vi "Pulse Gen Control Panel (No Objects).vi"(8 "error in (no error)":errorcluster) -> (0 "error out":errorcluster)   [LabVIEW 2009]
uses:
  Global/GPIB Numbers.vi
  Pulse Generator.lvclass
panel:
  in  "Width/Duty\nUP/DOWN Ch2":bool
  in  "Width/Duty\nUP/DOWN Ch1":bool
  in  "Clear Error":bool
  out "Ready when \nblinking":bool
  in  "Copy actual to set":bool
  out "Pulse Mode":enum16{"Pulses", "Pattern"}(ring)
  out "Arming (Trigger) Source":T1(ring)
  in  "Populate fields with member data":bool
  out "Strobe Pattern":string
  in  "Strobe Pattern Set":string
  out "StrobeDataBuffer":digitalwaveform(graph)
  in  "Enable/disable":bool
  in  "Modes (changes immediately)":T2(radio)
  in  "BitPeriodSet":dbl[unit]
  out "BitPeriod":dbl[unit]
  out "Ch2Pattern":string
  in  "Ch2Pattern Set":string
  out "Ch1Pattern":string
  in  "Set Patterns":bool
  in  "Ch1Pattern Set":string
  in  "Ch2Duty (%) Set":dbl=10.0
  in  "Ch1Duty (%) Set":dbl=10.0
  in  "Ch1Delay Set":dbl[unit]
  in  "Ch2Delay Set":dbl[unit]
  in  "stop":bool
  out "Ch1DataBuffer":digitalwaveform(graph)
  out "Ch2DataBuffer":digitalwaveform(graph)
  in  "Ch2 Sync":bool
  in  "Ch1 Sync":bool
  in  "Ch2 Toggle":bool
  in  "Ch1 NOT Toggle":bool
  in  "Ch1 Toggle":bool
  in  "Ch2 NOT Toggle":bool
  in  "OverallPeriodSet":dbl[unit]
  in  "Ch2WidthSet":dbl[unit]=1e-09
  in  "Ch1WidthSet":dbl[unit]=1e-09
  in  "Ch2LowSet":dbl[unit]
  in  "Ch2HighSet":dbl[unit]
  in  "Ch1LowSet":dbl[unit]
  in  "Ch1HighSet":dbl[unit]
  in  "OverallFreqSet":dbl[unit]
  in  "Read to Control":bool
  in  "Set":bool
  out "Ch2Duty (%)":dbl
  out "Ch1Duty (%)":dbl
  out "Ch1Delay":dbl[unit]
  out "Ch2Delay":dbl[unit]
  out "Ch1Low":dbl[unit]
  out "Ch1High":dbl[unit]
  out "Ch2Width":dbl[unit]
  out "Ch1Width":dbl[unit]
  out "OverallPeriod":dbl[unit]
  out "Ch2Low":dbl[unit]
  out "Ch2High":dbl[unit]
  in  "Read":bool
  out "OverallFreq":dbl[unit]
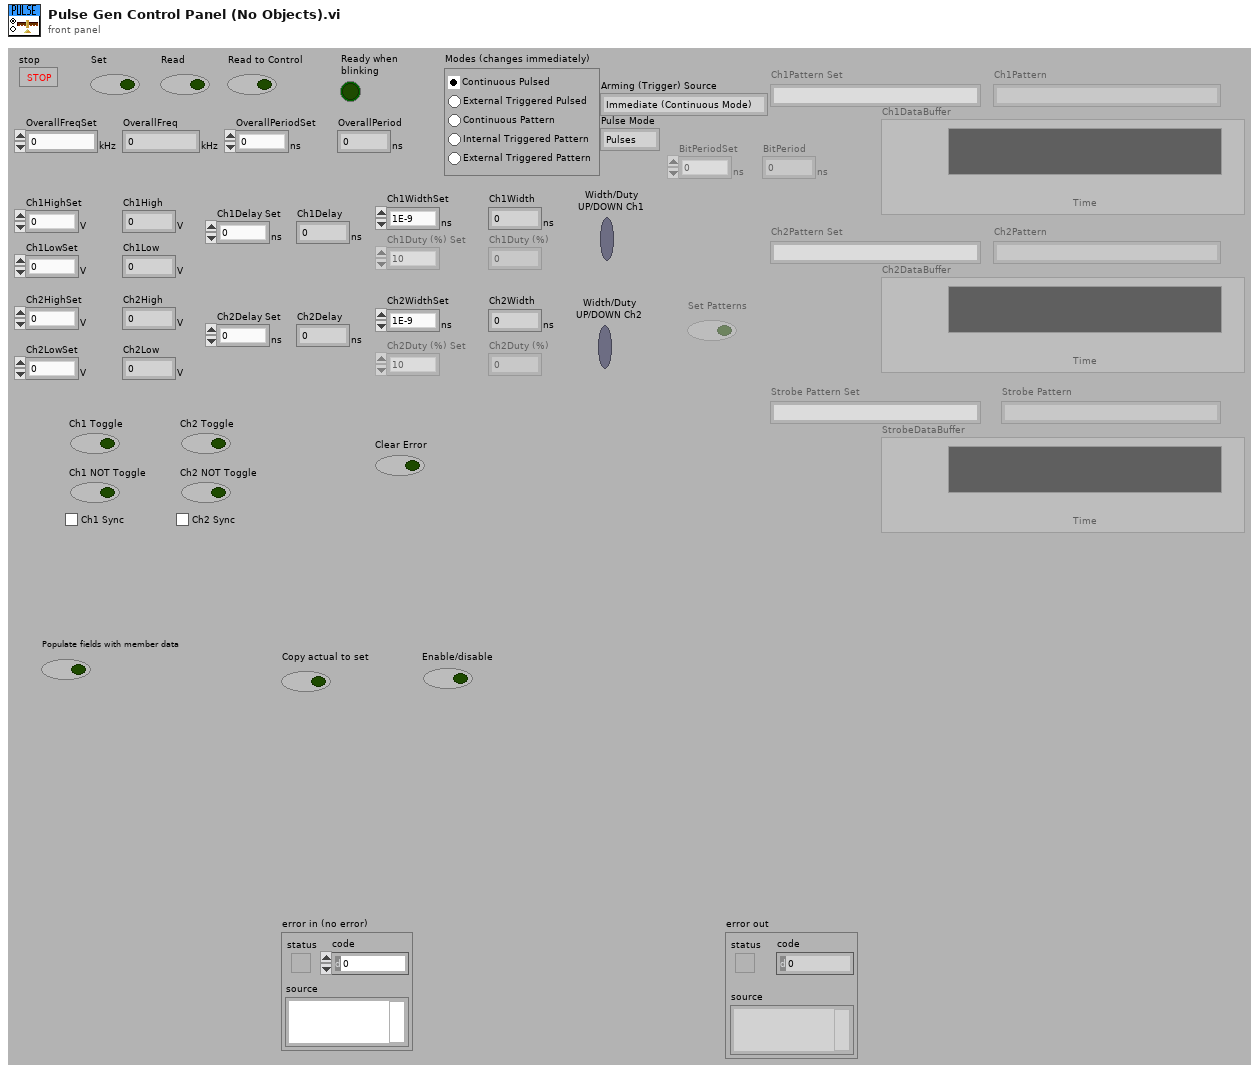
[diagram p1: front panel]
types:
  T1 = enum16{"Immediate (Continuous Mode)", "Internal PLL", "External", "Manual"}
  T2 = enum32{"Continuous Pulsed", "Continuous Pattern", "Internal Triggered Pattern", "External Triggered Pulsed", "External Triggered Pattern", "Other"}
  T3 = cluster{"Arming (Trigger) Source":u16, "Pulse Mode":u16, "Overall Period":dbl[unit], "Ch1Delay":dbl[unit], "Ch1Width":dbl[unit], "Ch2Delay":dbl[unit], "Ch2Width":dbl[unit], "Output Levels":cluster{"1 High":dbl[unit], "1 Low":dbl[unit], "2 High":dbl[unit], "2 Low":dbl[unit]}, "Outputs 1/!1/2/!2 ":bool[], "Bit Period":dbl[unit], "Ch1 Pattern":string, "Ch2 Pattern":string, "Strobe Pattern":string, "Ch1Width(true)":bool, "Ch2Width(true)":bool}
  T4 = typedef "GPIB Type Def.ctl" = cluster{"Name":string, "bus":dbl, "GPIB":dbl, "GPIB as string":string, "byte":i32, "VISA Resource Name":refnum<visa-resource-name>}
  T5 = enum16{"Internal Oscillator", "Internal PLL", "External Clock "}
  T6 = enum16{"Internal Oscillator", "Internal PLL", "Clock Input"}
  T7 = enum16{"Channel All ", "Channel 1", "Channel 2", "Channel 3", "Channels Combined"}
  T8 = cluster{"1 High":dbl[unit], "1 Low":dbl[unit], "2 High":dbl[unit], "2 Low":dbl[unit]}
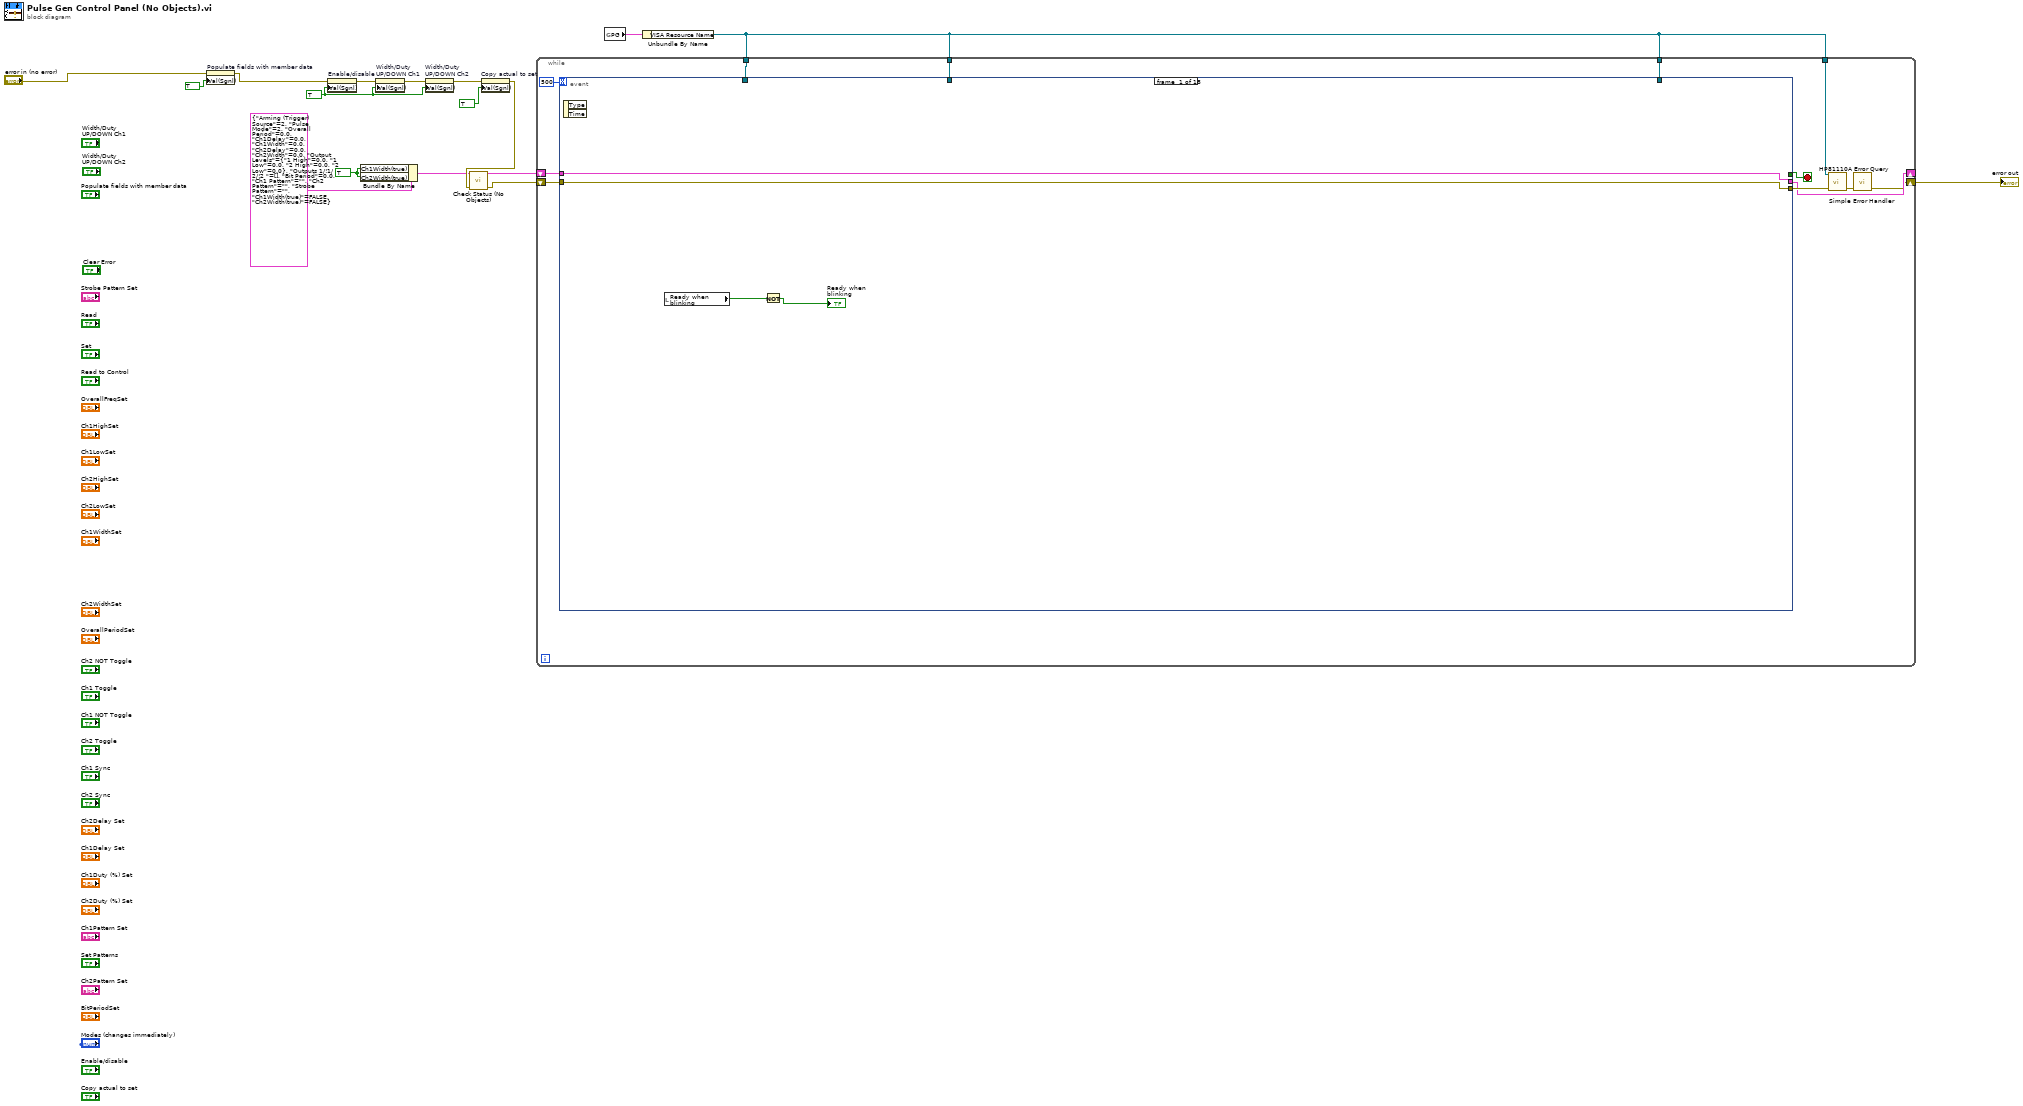
[diagram p0: block diagram]
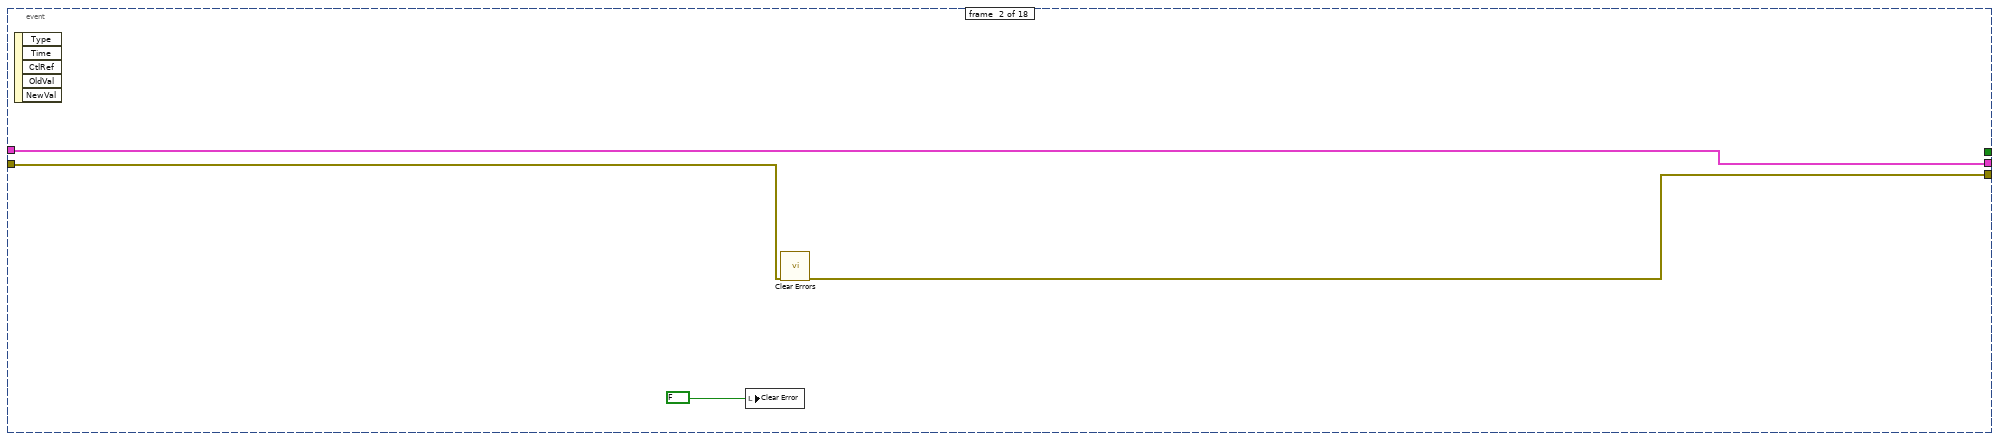
[diagram p2: hidden frame]
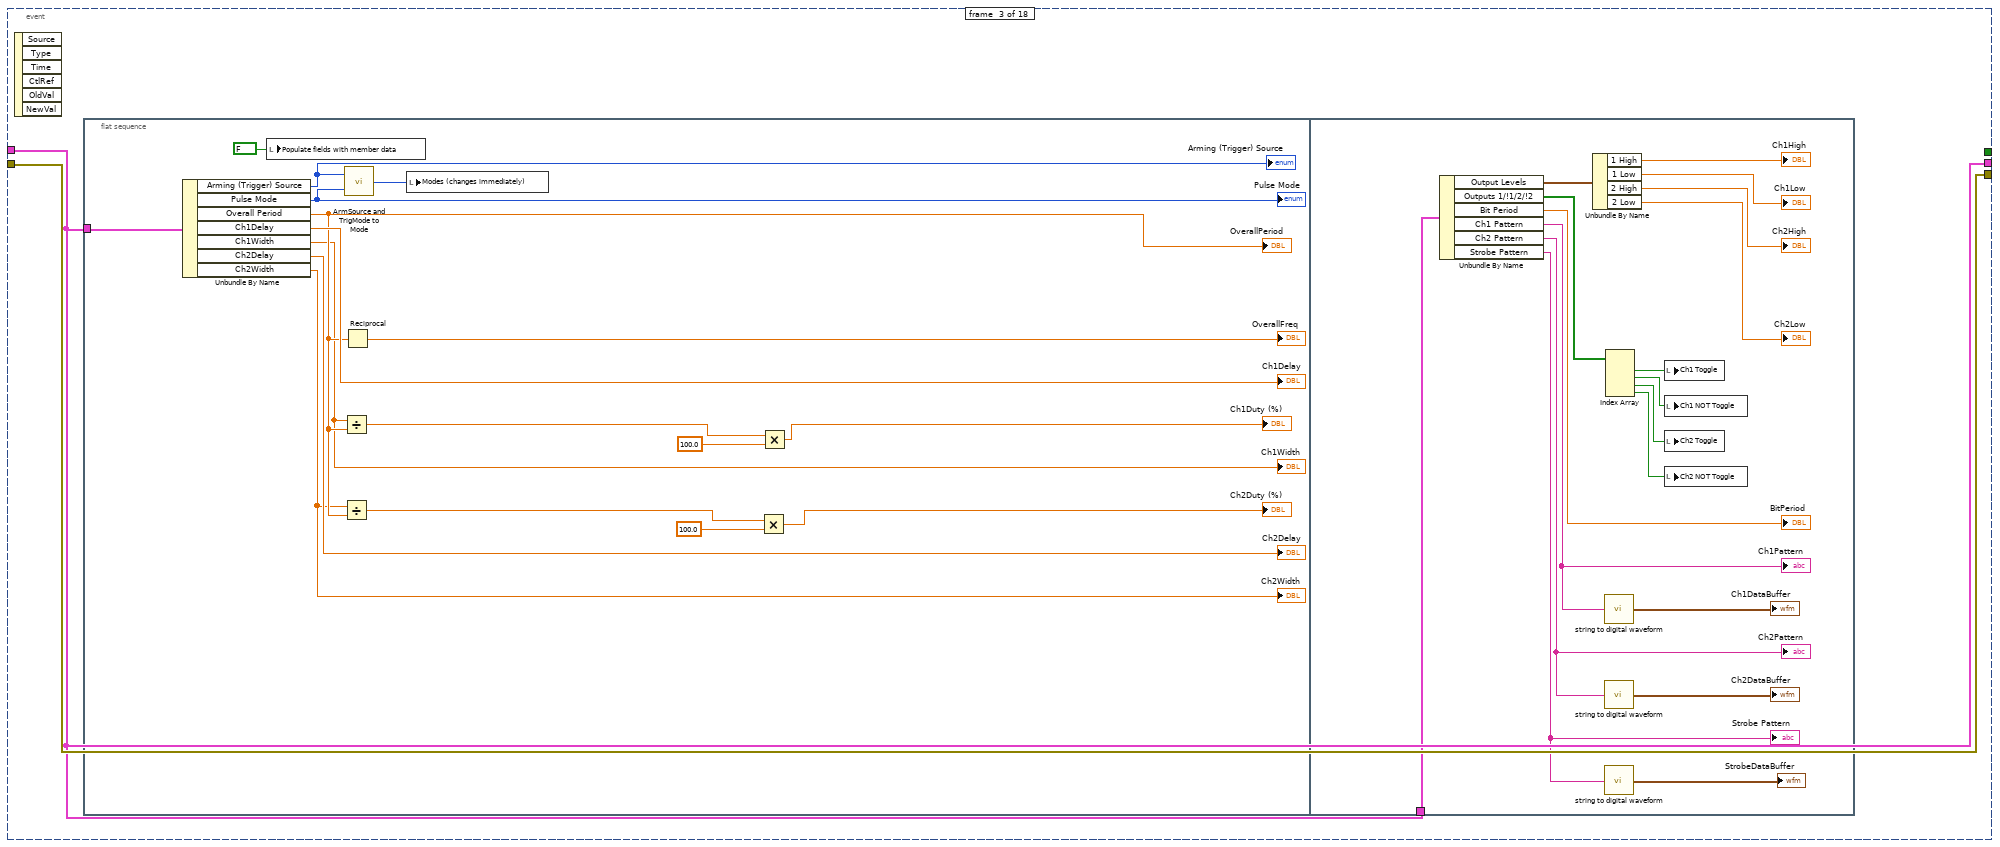
[diagram p3: hidden frame]
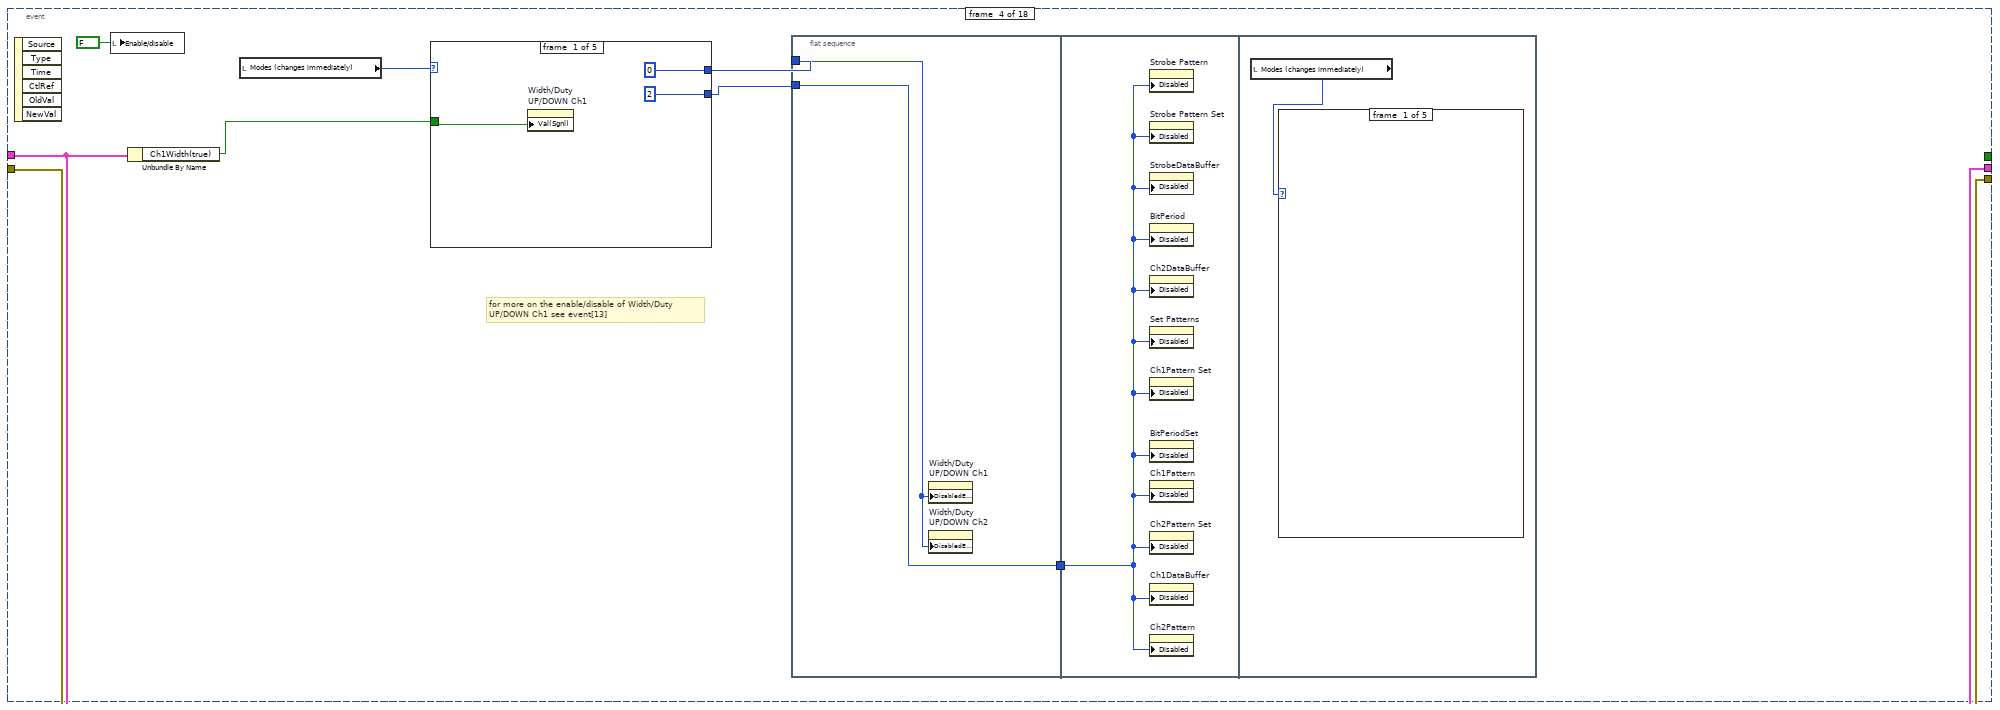
[diagram p4: hidden frame]
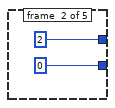
[diagram p5: hidden frame]
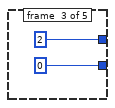
[diagram p6: hidden frame]
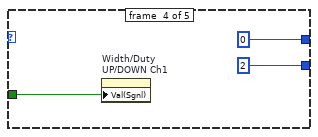
[diagram p7: hidden frame]
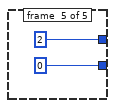
[diagram p8: hidden frame]
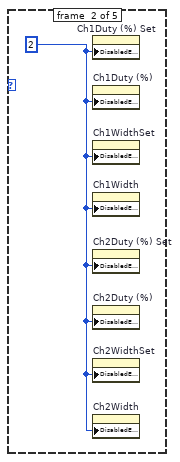
[diagram p9: hidden frame]
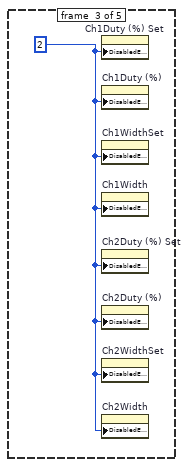
[diagram p10: hidden frame]
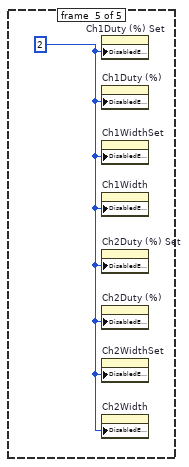
[diagram p12: hidden frame]
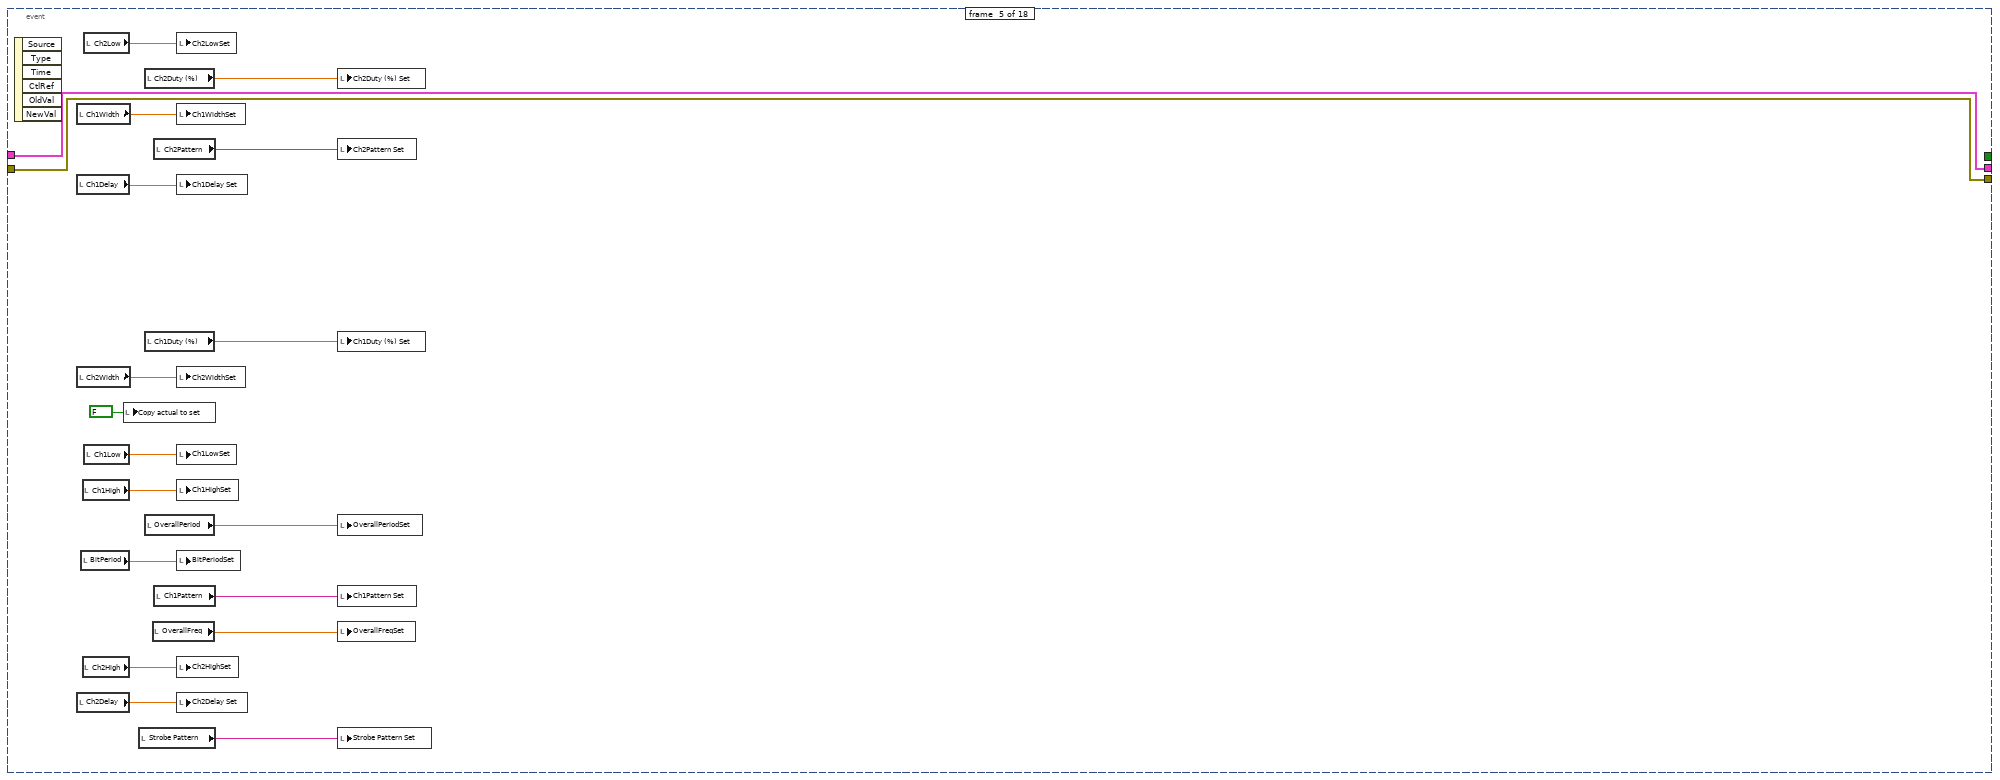
[diagram p13: hidden frame]
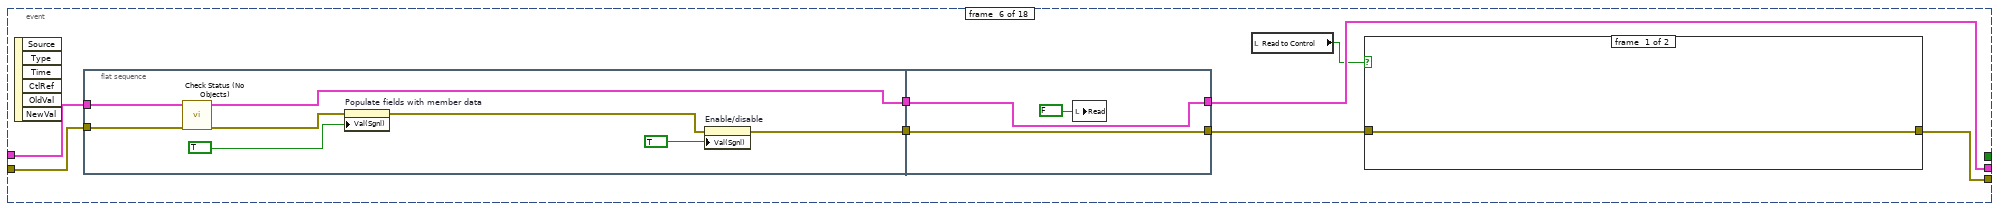
[diagram p14: hidden frame]
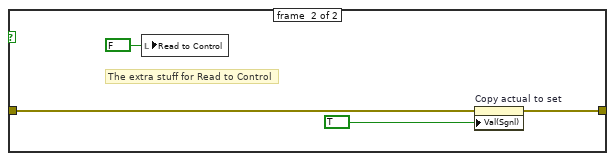
[diagram p15: hidden frame]
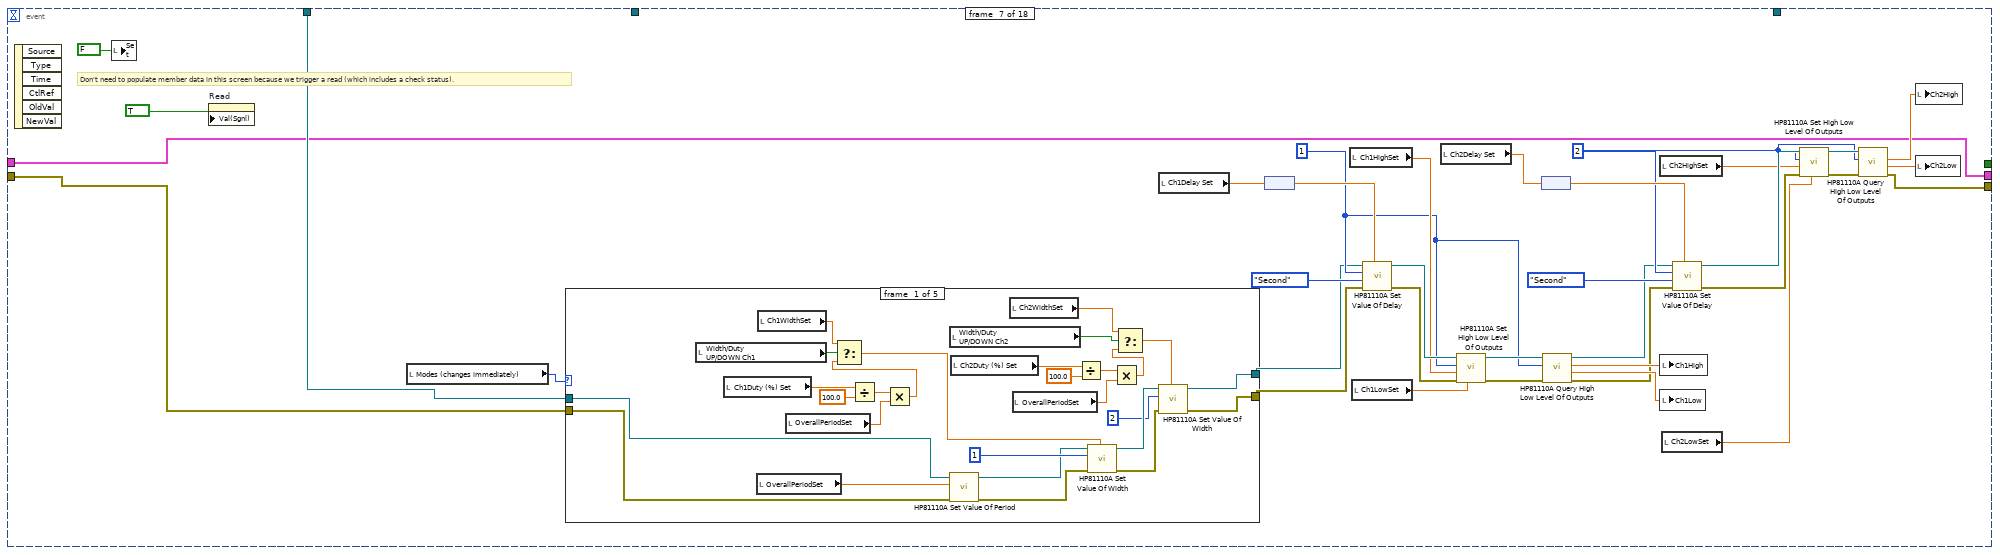
[diagram p16: hidden frame]
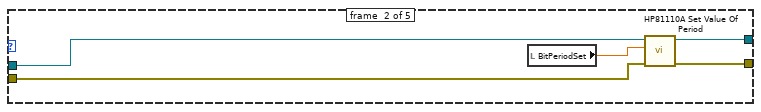
[diagram p17: hidden frame]
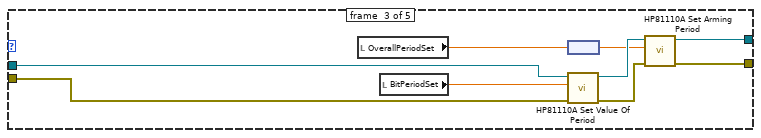
[diagram p18: hidden frame]
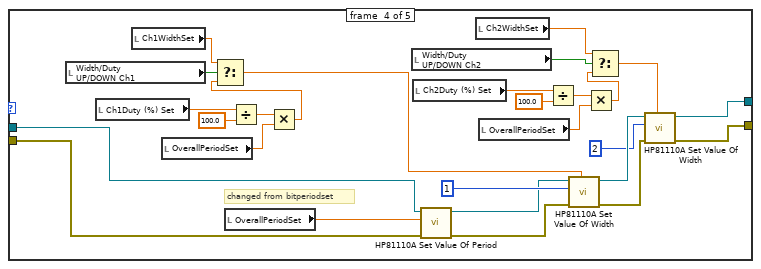
[diagram p19: hidden frame]
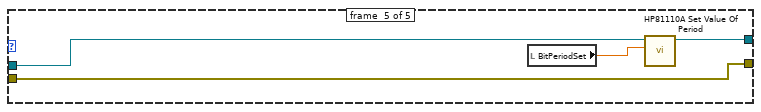
[diagram p20: hidden frame]
diagram:
  w10 = TRUE
  w11 = TRUE ("Value (Signaling)")
  n1 = property on="Populate fields with member data" class="Bool (strict)"(error in="error in (no error)", "Val(Sgnl)"=TRUE ("Value (Signaling)")) -> (error out=w15:errorcluster)  [unwired: 1 in, 1 out]
  n2 = property on="Enable/disable" class="Bool (strict)"(error in=w15, "Val(Sgnl)"=w11) -> (error out=w14:errorcluster)  [unwired: 1 in, 1 out]
  n3 = Bundle By Name(cluster=T3 {"Arming (Trigger) Source"=2, "Pulse Mode"=2, "Overall Period"=0.0, "Ch1Delay"=0.0, "Ch1Width"=0.0, "Ch2Delay"=0.0, "Ch2Width"=0.0, "Output Levels"={"1 High"=0.0, "1 Low"=0.0, "2 High"=0.0, "2 Low"=0.0}, "Outputs 1/!1/2/!2 "=[], "Bit Period"=0.0, "Ch1 Pattern"="", "Ch2 Pattern"="", "Strobe Pattern"="", "Ch1Width(true)"=FALSE, "Ch2Width(true)"=FALSE} ("Cluster of class private data"), "Ch1Width(true)"=w10, "Ch2Width(true)"=w10) -> (w1:T3)
  n4 = property on="Width/Duty\nUP/DOWN Ch1" class="Bool (strict)"(error in=w14, "Val(Sgnl)"=w11) -> (error out=w12:errorcluster)  [unwired: 1 in, 1 out]
  n5 = property on="Width/Duty\nUP/DOWN Ch2" class="Bool (strict)"(error in=w12, "Val(Sgnl)"=w11) -> (error out=w13:errorcluster)  [unwired: 1 in, 1 out]
  n6 = property on="Copy actual to set" class="Bool (strict)"(error in=w13, "Val(Sgnl)"=TRUE ("Value (Signaling)")) -> (error out=w4:errorcluster)  [unwired: 1 in, 1 out]
  n7 = call "Check Status (No Objects).vi"("error in (no error)"=w4, "Cluster In"=w1) -> ("error out"=w3:errorcluster, "Cluster Out"=w2:T3)  [unwired: 6 in, 2 out]
  n8 = global read "GPIB Numbers.vi" "PG"() -> (w7:T4)
  n9 = Unbundle By Name(w7) -> ("VISA Resource Name"=w5:refnum<visa-resource-name>)
  n10 = while {
    shift-right: [w22] -> _
    shift-left: w2 -> [w27]
    shift-right: [w18] -> w6
    shift-left: w3 -> [w26]
    tunnel: w5 -> [w24]
    tunnel: w5 -> [w21]
    tunnel: w5 -> [w20]
    tunnel: w5 -> [w19]
    stop <- w29 stop-if-true
    n11 = event shown="[5] \"Read\", \"Read to Control\": Value Change" {
      selector: _ -> [_ _ _ _ _ _ _ _ _ _ _ _ _ _ _ _ _ _]
      dyn-events: _ -> [_ _ _ _ _ _ _ _ _ _ _ _ _ _ _ _ _ _]
      timeout: 500 -> [_ _ _ _ _ _ _ _ _ _ _ _ _ _ _ _ _ _]
      tunnel: [_ _ _ _ _ _ _ _ _ _ _ _ "stop" _ _ _ _ _] -> w29
      tunnel: w26 -> [w32 w37 w39 w81 w103 w128 w147 w252 w280 w295 w314 w337 w350 w370 w372 w382 w392 w398]
      tunnel: [w32 w35 w39 w81 w103 w124 w146 w254 w282 w294 w314 w337 w350 w370 w372 w382 w392 w398] -> w23
      tunnel: w27 -> [w33 w36 w38 w76 w104 w127 w145 w253 w281 w293 w315 w338 w349 w357 w371 w381 w391 w399]
      tunnel: [w33 w36 w38 w76 w104 w126 w145 w253 w281 w302 w315 w338 w349 w356 w371 w381 w391 w399] -> w22
      tunnel: w21 -> [_ _ _ _ _ _ w148 _ _ _ _ _ _ _ _ _ _ _]
      tunnel: w20 -> [_ _ _ _ _ _ _ w255 w279 _ _ _ _ _ _ _ _ _]
      tunnel: w19 -> [_ _ _ _ _ _ _ _ _ w296 _ _ _ _ _ _ _ _]
      event #0 {
        n12 = event-data() -> ()  [unwired: 3 out]
        n13 = local read "Ready when \nblinking"() -> (w31:bool)
        n14 = Not(x=w31) -> (.not. x?=→"Ready when \nblinking":bool)
      }
      event #1 {
        n15 = event-data() -> ()  [unwired: 6 out]
        n16 = local write "Clear Error"(FALSE ("Clear Error")) -> ()
        n17 = call <vilib>:"Clear Errors.vi"("error in (no error)"=w37) -> ("error out"=w35:errorcluster)  [unwired: 6 in]
      }
      event #2 {
        n18 = event-data() -> ()  [unwired: 7 out]
        n19 = flat-sequence {
          tunnel: w38 -> [w46]
          tunnel: w38 -> [w57]
          frame #0 {
            n20 = Unbundle By Name(w46) -> ("Arming (Trigger) Source"=w49:u16, "Pulse Mode"=w48:u16, "Overall Period"=w52:dbl[unit], "Ch1Delay"=→"Ch1Delay":dbl[unit], "Ch1Width"=w51:dbl[unit], "Ch2Delay"=→"Ch2Delay":dbl[unit], "Ch2Width"=w50:dbl[unit])
            "OverallPeriod" <- w52
            "Ch1Width" <- w51
            "Ch2Width" <- w50
            "Arming (Trigger) Source" <- w49
            "Pulse Mode" <- w48
            n21 = local write "Populate fields with member data"(FALSE ("Populate fields with member data")) -> ()
            n22 = Divide(x=w51, y=w52) -> (x/y=w43:dbl)
            n23 = Divide(x=w50, y=w52) -> (x/y=w41:dbl)
            n24 = Reciprocal(x=w52) -> (1/x=→"OverallFreq":dbl[unit])
            n25 = call "ArmSource and TrigMode to Mode.vi"("Pulse Mode"=w48, "Arming (Trigger) Source (0:Internal PLL)"=w49) -> ("Modes (changes immediately)"=w47:T2)
            n26 = local write "Modes (changes immediately)"(w47) -> ()
            n27 = Multiply(x=w41, y=100.0) -> (x*y=→"Ch2Duty (%)":dbl)
            n28 = Multiply(x=w43, y=100.0) -> (x*y=→"Ch1Duty (%)":dbl)
          }
          frame #1 {
            n29 = Unbundle By Name(w57) -> ("Output Levels"=w69:T8, "Outputs 1/!1/2/!2"=w70:bool[], "Bit Period"=→"BitPeriod":dbl[unit], "Ch1 Pattern"=w72:string, "Ch2 Pattern"=w73:string, "Strobe Pattern"=w74:string)
            "Ch1Pattern" <- w72
            "Ch2Pattern" <- w73
            "Strobe Pattern" <- w74
            n30 = Unbundle By Name(w69) -> ("1 High"=→"Ch1High":dbl[unit], "1 Low"=→"Ch1Low":dbl[unit], "2 High"=→"Ch2High":dbl[unit], "2 Low"=→"Ch2Low":dbl[unit])
            n31 = call "string to digital waveform.vi"("String"=w72) -> ("digital waveform"=→"Ch1DataBuffer":digitalwaveform)
            n32 = call "string to digital waveform.vi"("String"=w73) -> ("digital waveform"=→"Ch2DataBuffer":digitalwaveform)
            n33 = call "string to digital waveform.vi"("String"=w74) -> ("digital waveform"=→"StrobeDataBuffer":digitalwaveform)
            n34 = Index Array(array=w70) -> (element #1=w65:bool, element #2=w66:bool, element #3=w67:bool, element #4=w68:bool)  [unwired: 4 in]
            n35 = local write "Ch1 Toggle"(w65) -> ()
            n36 = local write "Ch1 NOT Toggle"(w66) -> ()
            n37 = local write "Ch2 Toggle"(w67) -> ()
            n38 = local write "Ch2 NOT Toggle"(w68) -> ()
          }
        }
      }
      event #3 {
        # "for more on the enable/disable of Width/Duty\nUP/DOWN Ch1 see event[13]"
        n39 = event-data() -> ()  [unwired: 7 out]
        n40 = local write "Enable/disable"(FALSE ("Enable/disable")) -> ()
        n41 = Unbundle By Name(w76) -> ("Ch1Width(true)"=w75:bool)
        n42 = local read "Modes (changes immediately)"() -> (w79:T2)
        n43 = case shown="\"Internal Triggered Pattern\"" w79 {
          tunnel: [2 0 0 2 0] -> w77
          tunnel: [0 2 2 0 2] -> w78
          tunnel: w75 -> [w83 _ _ w90 _]
          frame #0 {
            n44 = property on="Width/Duty\nUP/DOWN Ch1" class="Bool (strict)"("Val(Sgnl)"=w83) -> ()  [unwired: 2 in, 2 out]
          }
          frame #1 {
          }
          frame #2 {
          }
          frame #3 {
            n45 = property on="Width/Duty\nUP/DOWN Ch1" class="Bool (strict)"("Val(Sgnl)"=w90) -> ()  [unwired: 2 in, 2 out]
          }
          frame #4 {
          }
        }
        n46 = flat-sequence {
          tunnel: [w96] -> w80
          tunnel: w78 -> [w95]
          tunnel: w77 -> [w96]
          tunnel: w80 -> [w97]
          frame #0 {
            n47 = property on="Width/Duty\nUP/DOWN Ch1" class="Bool (strict)"("DisabledEnum"=w95) -> ()  [unwired: 2 in, 2 out]
            n48 = property on="Width/Duty\nUP/DOWN Ch2" class="Bool (strict)"("DisabledEnum"=w95) -> ()  [unwired: 2 in, 2 out]
          }
          frame #1 {
            n49 = property on="Strobe Pattern" class="Str"("Disabled"=w97) -> ()  [unwired: 2 in, 2 out]
            n50 = property on="Strobe Pattern Set" class="Str"("Disabled"=w97) -> ()  [unwired: 2 in, 2 out]
            n51 = property on="StrobeDataBuffer" class="DigitalGraph (strict)"("Disabled"=w97) -> ()  [unwired: 2 in, 2 out]
            n52 = property on="BitPeriod" class="DigNum (strict)"("Disabled"=w97) -> ()  [unwired: 2 in, 2 out]
            n53 = property on="Ch2DataBuffer" class="DigitalGraph (strict)"("Disabled"=w97) -> ()  [unwired: 2 in, 2 out]
            n54 = property on="Set Patterns" class="Bool (strict)"("Disabled"=w97) -> ()  [unwired: 2 in, 2 out]
            n55 = property on="Ch1Pattern Set" class="Str"("Disabled"=w97) -> ()  [unwired: 2 in, 2 out]
            n56 = property on="BitPeriodSet" class="DigNum (strict)"("Disabled"=w97) -> ()  [unwired: 2 in, 2 out]
            n57 = property on="Ch1Pattern" class="Str"("Disabled"=w97) -> ()  [unwired: 2 in, 2 out]
            n58 = property on="Ch2Pattern Set" class="Str"("Disabled"=w97) -> ()  [unwired: 2 in, 2 out]
            n59 = property on="Ch1DataBuffer" class="DigitalGraph (strict)"("Disabled"=w97) -> ()  [unwired: 2 in, 2 out]
            n60 = property on="Ch2Pattern" class="Str"("Disabled"=w97) -> ()  [unwired: 2 in, 2 out]
          }
          frame #2 {
            n61 = local read "Modes (changes immediately)"() -> (w98:T2)
            n62 = case shown="\"External Triggered Pattern\"" w98 {
              frame #0 {
              }
              frame #1 {
                w99 = 2
                n63 = property on="Ch1Duty (%) Set" class="DigNum (strict)"("DisabledEnum"=w99) -> ()  [unwired: 2 in, 2 out]
                n64 = property on="Ch1Duty (%)" class="DigNum (strict)"("DisabledEnum"=w99) -> ()  [unwired: 2 in, 2 out]
                n65 = property on="Ch1WidthSet" class="DigNum (strict)"("DisabledEnum"=w99) -> ()  [unwired: 2 in, 2 out]
                n66 = property on="Ch1Width" class="DigNum (strict)"("DisabledEnum"=w99) -> ()  [unwired: 2 in, 2 out]
                n67 = property on="Ch2Duty (%) Set" class="DigNum (strict)"("DisabledEnum"=w99) -> ()  [unwired: 2 in, 2 out]
                n68 = property on="Ch2Duty (%)" class="DigNum (strict)"("DisabledEnum"=w99) -> ()  [unwired: 2 in, 2 out]
                n69 = property on="Ch2WidthSet" class="DigNum (strict)"("DisabledEnum"=w99) -> ()  [unwired: 2 in, 2 out]
                n70 = property on="Ch2Width" class="DigNum (strict)"("DisabledEnum"=w99) -> ()  [unwired: 2 in, 2 out]
              }
              frame #2 {
                w100 = 2
                n71 = property on="Ch1Duty (%) Set" class="DigNum (strict)"("DisabledEnum"=w100) -> ()  [unwired: 2 in, 2 out]
                n72 = property on="Ch1Duty (%)" class="DigNum (strict)"("DisabledEnum"=w100) -> ()  [unwired: 2 in, 2 out]
                n73 = property on="Ch1WidthSet" class="DigNum (strict)"("DisabledEnum"=w100) -> ()  [unwired: 2 in, 2 out]
                n74 = property on="Ch1Width" class="DigNum (strict)"("DisabledEnum"=w100) -> ()  [unwired: 2 in, 2 out]
                n75 = property on="Ch2Duty (%) Set" class="DigNum (strict)"("DisabledEnum"=w100) -> ()  [unwired: 2 in, 2 out]
                n76 = property on="Ch2Duty (%)" class="DigNum (strict)"("DisabledEnum"=w100) -> ()  [unwired: 2 in, 2 out]
                n77 = property on="Ch2WidthSet" class="DigNum (strict)"("DisabledEnum"=w100) -> ()  [unwired: 2 in, 2 out]
                n78 = property on="Ch2Width" class="DigNum (strict)"("DisabledEnum"=w100) -> ()  [unwired: 2 in, 2 out]
              }
              frame #3 {
              }
              frame #4 {
                w101 = 2
                n79 = property on="Ch1Duty (%) Set" class="DigNum (strict)"("DisabledEnum"=w101) -> ()  [unwired: 2 in, 2 out]
                n80 = property on="Ch1Duty (%)" class="DigNum (strict)"("DisabledEnum"=w101) -> ()  [unwired: 2 in, 2 out]
                n81 = property on="Ch1WidthSet" class="DigNum (strict)"("DisabledEnum"=w101) -> ()  [unwired: 2 in, 2 out]
                n82 = property on="Ch1Width" class="DigNum (strict)"("DisabledEnum"=w101) -> ()  [unwired: 2 in, 2 out]
                n83 = property on="Ch2Duty (%) Set" class="DigNum (strict)"("DisabledEnum"=w101) -> ()  [unwired: 2 in, 2 out]
                n84 = property on="Ch2Duty (%)" class="DigNum (strict)"("DisabledEnum"=w101) -> ()  [unwired: 2 in, 2 out]
                n85 = property on="Ch2WidthSet" class="DigNum (strict)"("DisabledEnum"=w101) -> ()  [unwired: 2 in, 2 out]
                n86 = property on="Ch2Width" class="DigNum (strict)"("DisabledEnum"=w101) -> ()  [unwired: 2 in, 2 out]
              }
            }
          }
        }
      }
      event #4 {
        n87 = event-data() -> ()  [unwired: 7 out]
        n88 = local read "Ch1Width"() -> (w116:dbl[unit])
        n89 = local read "Ch1Delay"() -> (w114:dbl[unit])
        n90 = local read "Ch2Width"() -> (w112:dbl[unit])
        n91 = local read "Ch2Delay"() -> (w110:dbl[unit])
        n92 = local read "BitPeriod"() -> (w106:dbl[unit])
        n93 = local read "Ch1High"() -> (w118:dbl[unit])
        n94 = local read "Ch2High"() -> (w109:dbl[unit])
        n95 = local read "Ch2Low"() -> (w113:dbl[unit])
        n96 = local read "Ch1Low"() -> (w117:dbl[unit])
        n97 = local write "Copy actual to set"(FALSE ("Copy actual to set")) -> ()
        n98 = local read "Strobe Pattern"() -> (w102:string)
        n99 = local read "Ch2Duty (%)"() -> (w111:dbl)
        n100 = local read "Ch1Duty (%)"() -> (w115:dbl)
        n101 = local read "OverallPeriod"() -> (w119:dbl[unit])
        n102 = local read "OverallFreq"() -> (w120:dbl[unit])
        n103 = local read "Ch2Pattern"() -> (w107:string)
        n104 = local read "Ch1Pattern"() -> (w108:string)
        n105 = local write "Ch2LowSet"(w113) -> ()
        n106 = local write "Ch1WidthSet"(w116) -> ()
        n107 = local write "Ch1Delay Set"(w114) -> ()
        n108 = local write "Ch2WidthSet"(w112) -> ()
        n109 = local write "Ch1LowSet"(w117) -> ()
        n110 = local write "Ch1HighSet"(w118) -> ()
        n111 = local write "BitPeriodSet"(w106) -> ()
        n112 = local write "Ch2HighSet"(w109) -> ()
        n113 = local write "Ch2Delay Set"(w110) -> ()
        n114 = local write "Ch2Duty (%) Set"(w111) -> ()
        n115 = local write "Ch2Pattern Set"(w107) -> ()
        n116 = local write "Ch1Duty (%) Set"(w115) -> ()
        n117 = local write "OverallPeriodSet"(w119) -> ()
        n118 = local write "Ch1Pattern Set"(w108) -> ()
        n119 = local write "OverallFreqSet"(w120) -> ()
        n120 = local write "Strobe Pattern Set"(w102) -> ()
      }
      event #5 {
        n121 = event-data() -> ()  [unwired: 7 out]
        n122 = flat-sequence {
          tunnel: w128 -> [w136]
          tunnel: w127 -> [w129]
          tunnel: [w135] -> w122
          tunnel: [w134] -> w121
          tunnel: [w138] -> w125
          tunnel: [w139] -> w126
          tunnel: w122 -> [w139]
          tunnel: w121 -> [w138]
          frame #0 {
            n123 = call "Check Status (No Objects).vi"("error in (no error)"=w136, "Cluster In"=w129) -> ("error out"=w131:errorcluster, "Cluster Out"=w135:T3)  [unwired: 6 in, 2 out]
            n124 = property on="Populate fields with member data" class="Bool (strict)"(error in=w131, "Val(Sgnl)"=TRUE ("Value (Signaling)")) -> (error out=w130:errorcluster)  [unwired: 1 in, 1 out]
            n125 = property on="Enable/disable" class="Bool (strict)"(error in=w130, "Val(Sgnl)"=TRUE ("Value (Signaling)")) -> (error out=w134:errorcluster)  [unwired: 1 in, 1 out]
          }
          frame #1 {
            n126 = local write "Read"(FALSE) -> ()
          }
        }
        n127 = local read "Read to Control"() -> (w123:bool)
        n128 = case shown="False" w123 {
          tunnel: w125 -> [w140 w142]
          tunnel: [w140 w141] -> w124
          frame #0 {
          }
          frame #1 {
            # "The extra stuff for Read to Control"
            n129 = local write "Read to Control"(FALSE) -> ()
            n130 = property on="Copy actual to set" class="Bool (strict)"(error in=w142, "Val(Sgnl)"=TRUE ("Value (Signaling)")) -> (error out=w141:errorcluster)  [unwired: 1 in, 1 out]
          }
        }
      }
      event #6 {
        w154 = 1
        w159 = 2
        # "Don't need to populate member data in this screen because we trigger a read (which includes a check status)."
        n131 = event-data() -> ()  [unwired: 7 out]
        n132 = local write "Set"(FALSE) -> ()
        n133 = property on="Read" class="Bool (strict)"("Val(Sgnl)"=TRUE ("Value (Signaling)")) -> ()  [unwired: 2 in, 2 out]
        n134 = local read "Modes (changes immediately)"() -> (w151:T2)
        n135 = case shown="\"External Triggered Pulsed\"" w151 {
          tunnel: w148 -> [w201 w210 w215 w221 w250]
          tunnel: w147 -> [w200 w208 w213 w240 w248]
          tunnel: [w197 w209 w214 w241 w249] -> w150
          tunnel: [w196 w207 w212 w238 w248] -> w149
          frame #0 {
            n136 = local read "Width/Duty\nUP/DOWN Ch1"() -> (w195:bool)
            n137 = local read "Ch1Duty (%) Set"() -> (w192:dbl)
            n138 = local read "OverallPeriodSet"() -> (w206:dbl[unit])
            n139 = local read "Ch1WidthSet"() -> (w194:dbl[unit])
            n140 = local read "OverallPeriodSet"() -> (w190:dbl[unit])
            n141 = Divide(x=w192, y=100.0) -> (x/y=w191:dbl)
            n142 = Multiply(x=w191, y=w190) -> (x*y=w189:dbl[unit])
            n143 = Select(t=w194, s=w195, f=w189) -> (s? t:f=w180:dbl[unit])
            n144 = local read "Width/Duty\nUP/DOWN Ch2"() -> (w183:bool)
            n145 = call "HP81110A Set Value Of Period.vi"("error in (no error)"=w200, "Period Value"=w206, "VISA session"=w201) -> ("error out"=w198:errorcluster, "dup VISA session"=w199:refnum<visa-resource-name>)  [unwired: 7 out]
            n146 = local read "Ch2Duty (%) Set"() -> (w186:dbl)
            n147 = local read "Ch2WidthSet"() -> (w182:dbl[unit])
            n148 = local read "OverallPeriodSet"() -> (w188:dbl[unit])
            n149 = Divide(x=w186, y=100.0) -> (x/y=w187:dbl)
            n150 = call "HP81110A Set Value Of Width.vi"("Width Value (100.0E-9)"=w180, "error in (no error)"=w198, "Channel (1:Channel 1)"=1, "VISA session"=w199) -> ("error out"=w205:errorcluster, "dup VISA session"=w204:refnum<visa-resource-name>)  [unwired: 1 in, 5 out]
            n151 = Multiply(x=w187, y=w188) -> (x*y=w184:dbl[unit])
            n152 = Select(t=w182, s=w183, f=w184) -> (s? t:f=w181:dbl[unit])
            n153 = call "HP81110A Set Value Of Width.vi"("Width Value (100.0E-9)"=w181, "error in (no error)"=w205, "Channel (1:Channel 1)"=2, "VISA session"=w204) -> ("error out"=w196:errorcluster, "dup VISA session"=w197:refnum<visa-resource-name>)  [unwired: 1 in, 5 out]
          }
          frame #1 {
            n154 = local read "BitPeriodSet"() -> (w211:dbl[unit])
            n155 = call "HP81110A Set Value Of Period.vi"("error in (no error)"=w208, "Period Value"=w211, "VISA session"=w210) -> ("error out"=w207:errorcluster, "dup VISA session"=w209:refnum<visa-resource-name>)  [unwired: 7 out]
          }
          frame #2 {
            n156 = local read "OverallPeriodSet"() -> (w217:dbl[unit])
            n157 = local read "BitPeriodSet"() -> (w216:dbl[unit])
            n158 = node(w217) -> (w218:dbl)
            n159 = call "HP81110A Set Value Of Period.vi"("error in (no error)"=w213, "Period Value"=w216, "VISA session"=w215) -> ("error out"=w220:errorcluster, "dup VISA session"=w219:refnum<visa-resource-name>)  [unwired: 7 out]
            n160 = call "HP81110A Set Arming Period.vi"("error in (no error)"=w220, "Period Value (10.0E-6 Sec)"=w218, "VISA session"=w219) -> ("error out"=w212:errorcluster, "dup VISA session"=w214:refnum<visa-resource-name>)  [unwired: 7 out]
          }
          frame #3 {
            # "changed from bitperiodset"
            n161 = local read "Width/Duty\nUP/DOWN Ch1"() -> (w237:bool)
            n162 = local read "Ch1Duty (%) Set"() -> (w234:dbl)
            n163 = local read "Ch1WidthSet"() -> (w236:dbl[unit])
            n164 = local read "OverallPeriodSet"() -> (w232:dbl[unit])
            n165 = local read "OverallPeriodSet"() -> (w243:dbl[unit])
            n166 = Divide(x=w234, y=100.0) -> (x/y=w233:dbl)
            n167 = Multiply(x=w233, y=w232) -> (x*y=w231:dbl[unit])
            n168 = Select(t=w236, s=w237, f=w231) -> (s? t:f=w224:dbl[unit])
            n169 = local read "Width/Duty\nUP/DOWN Ch2"() -> (w226:bool)
            n170 = local read "Ch2Duty (%) Set"() -> (w228:dbl)
            n171 = call "HP81110A Set Value Of Period.vi"("error in (no error)"=w240, "Period Value"=w243, "VISA session"=w221) -> ("error out"=w239:errorcluster, "dup VISA session"=w242:refnum<visa-resource-name>)  [unwired: 7 out]
            n172 = local read "Ch2WidthSet"() -> (w225:dbl[unit])
            n173 = local read "OverallPeriodSet"() -> (w230:dbl[unit])
            n174 = Divide(x=w228, y=100.0) -> (x/y=w229:dbl)
            n175 = call "HP81110A Set Value Of Width.vi"("Width Value (100.0E-9)"=w224, "error in (no error)"=w239, "Channel (1:Channel 1)"=1, "VISA session"=w242) -> ("error out"=w247:errorcluster, "dup VISA session"=w246:refnum<visa-resource-name>)  [unwired: 1 in, 5 out]
            n176 = Multiply(x=w229, y=w230) -> (x*y=w222:dbl[unit])
            n177 = Select(t=w225, s=w226, f=w222) -> (s? t:f=w223:dbl[unit])
            n178 = call "HP81110A Set Value Of Width.vi"("Width Value (100.0E-9)"=w223, "error in (no error)"=w247, "Channel (1:Channel 1)"=2, "VISA session"=w246) -> ("error out"=w238:errorcluster, "dup VISA session"=w241:refnum<visa-resource-name>)  [unwired: 1 in, 5 out]
          }
          frame #4 {
            n179 = local read "BitPeriodSet"() -> (w251:dbl[unit])
            n180 = call "HP81110A Set Value Of Period.vi"("Period Value"=w251, "VISA session"=w250) -> ("dup VISA session"=w249:refnum<visa-resource-name>)  [unwired: 1 in, 8 out]
          }
        }
        n181 = local read "Ch1Delay Set"() -> (w177:dbl[unit])
        n182 = node(w177) -> (w176:dbl)
        n183 = local read "Ch1HighSet"() -> (w163:dbl[unit])
        n184 = local read "Ch1LowSet"() -> (w162:dbl[unit])
        n185 = call "HP81110A Set Value Of Delay.vi"("Delay Value (0.0)"=w176, "error in (no error)"=w149, "Delay Unit (0:Second)"=enum16{"Second", "Percent", "Degree", "Radians"}."Second", "Channel (1:Channel 1)"=w154, "VISA session"=w150) -> ("error out"=w167:errorcluster, "dup VISA session"=w166:refnum<visa-resource-name>)  [unwired: 5 out]
        n186 = local read "Ch2Delay Set"() -> (w175:dbl[unit])
        n187 = call "HP81110A Set High Low Level Of Outputs.vi"("Value Low (-0.5 V)"=w162, "error in (no error)"=w167, "Value High (0.5 V)"=w163, "Channel (1:Channel 1)"=w154, "VISA session"=w166) -> ("error out"=w164:errorcluster, "dup VISA session"=w165:refnum<visa-resource-name>)  [unwired: 5 out]
        n188 = node(w175) -> (w174:dbl)
        n189 = call "HP81110A Query High Low Level Of Outputs.vi"("error in (no error)"=w164, "Channel (1:Channel 1)"=w154, "VISA session"=w165) -> ("error out"=w152:errorcluster, "Value Low"=w160:dbl[unit], "Value High"=w161:dbl[unit], "dup VISA session"=w153:refnum<visa-resource-name>)  [unwired: 5 out]
        n190 = local read "Ch2HighSet"() -> (w158:dbl[unit])
        n191 = local write "Ch1High"(w161) -> ()
        n192 = local write "Ch1Low"(w160) -> ()
        n193 = local read "Ch2LowSet"() -> (w157:dbl[unit])
        n194 = call "HP81110A Set Value Of Delay.vi"("Delay Value (0.0)"=w174, "error in (no error)"=w152, "Delay Unit (0:Second)"=enum16{"Second", "Percent", "Degree", "Radians"}."Second", "Channel (1:Channel 1)"=w159, "VISA session"=w153) -> ("error out"=w169:errorcluster, "dup VISA session"=w171:refnum<visa-resource-name>)  [unwired: 5 out]
        n195 = call "HP81110A Set High Low Level Of Outputs.vi"("Value Low (-0.5 V)"=w157, "error in (no error)"=w169, "Value High (0.5 V)"=w158, "Channel (1:Channel 1)"=w159, "VISA session"=w171) -> ("error out"=w168:errorcluster, "dup VISA session"=w170:refnum<visa-resource-name>)  [unwired: 5 out]
        n196 = call "HP81110A Query High Low Level Of Outputs.vi"("error in (no error)"=w168, "Channel (1:Channel 1)"=w159, "VISA session"=w170) -> ("error out"=w146:errorcluster, "Value Low"=w155:dbl[unit], "Value High"=w156:dbl[unit])  [unwired: 6 out]
        n197 = local write "Ch2High"(w156) -> ()
        n198 = local write "Ch2Low"(w155) -> ()
      }
      event #7 {
        # "Don't need to populate member data in this screen because we trigger a read (which includes a check status)."
        n199 = event-data() -> ("NewVal"=w258:T2)  [unwired: 6 out]
        n200 = property on="Enable/disable" class="Bool (strict)"("Val(Sgnl)"=TRUE ("Value (Signaling)")) -> ()  [unwired: 2 in, 2 out]
        n201 = property on="Read" class="Bool (strict)"("Val(Sgnl)"=TRUE ("Value (Signaling)")) -> ()  [unwired: 2 in, 2 out]
        n202 = case shown="\"Continuous Pattern\"" w258 {
          tunnel: w252 -> [w261 w266 w269 w273 w276]
          tunnel: [w260 w265 w268 w272 w275] -> w254
          tunnel: w255 -> [w259 w263 w267 w271 w274]
          frame #0 {
            n203 = call "HP81110A Generating Cont Pulses.vi"("error in (no error)"=w261, "Period Source (0:Internal)"=T5."Internal Oscillator", "VISA session"=w259) -> ("error out"=w260:errorcluster)  [unwired: 1 in, 7 out]
          }
          frame #1 {
            n204 = call "HP81110A Generating Cont Pattern.vi"("error in (no error)"=w266, "Period Source (0:Internal Oscillator)"=T6."Internal Oscillator", "VISA session"=w263) -> ("error out"=w265:errorcluster)  [unwired: 1 in, 7 out]
          }
          frame #2 {
            n205 = call "HP81110A Generating Trigg Pattern.vi"("VISA session"=w267, "Trigger Source (0:Internal PLL)"=enum16{"Internal PLL", "External", "Manual"}."Internal PLL", "error in (no error)"=w269) -> ("error out"=w268:errorcluster)  [unwired: 5 in, 7 out]
          }
          frame #3 {
            n206 = call "HP81110A Generating Trigg Pulses.vi"("error in (no error)"=w273, "VISA session"=w271) -> ("error out"=w272:errorcluster)  [unwired: 2 in, 7 out]
          }
          frame #4 {
            n207 = call "HP81110A Generating Trigg Pattern.vi"("VISA session"=w274, "Period Source (0:Internal Oscillator)"=T6."Internal Oscillator", "Trigger Source (0:Internal PLL)"=enum16{"Internal PLL", "External", "Manual"}."External", "error in (no error)"=w276) -> ("error out"=w275:errorcluster)  [unwired: 4 in, 7 out]
          }
        }
      }
      event #8 {
        # "Don't need to populate member data in this screen because we trigger a read (which includes a check status)."
        n208 = event-data() -> ()  [unwired: 7 out]
        n209 = local write "Set Patterns"(FALSE) -> ()
        n210 = property on="Read" class="Bool (strict)"("Val(Sgnl)"=TRUE ("Value (Signaling)")) -> ()  [unwired: 2 in, 2 out]
        n211 = local read "Strobe Pattern Set"() -> (w284:string)
        n212 = local read "Ch1Pattern Set"() -> (w286:string)
        n213 = local read "Ch2Pattern Set"() -> (w285:string)
        n214 = call "three string merge.vi"("Strobe String (def: 10)"=w284, "Ch2 String"=w285, "Ch1 String"=w286) -> ("Merged Output String"=w283:string)  [unwired: 8 out]
        n215 = call "HP81110A Transfer String Into Memory.vi"("error in (no error)"=w280, "String"=w283, "Channel (1:Channel 1)"=T7."Channels Combined", "VISA session"=w279) -> ("error out"=w287:errorcluster, "dup VISA session"=w288:refnum<visa-resource-name>)  [unwired: 6 out]
        n216 = call "HP81110A Set Update Mode Of Pattern Data.vi"("error in (no error)"=w287, "Pattern Update Mode (1:Continuous)"=enum16{"Off", "Continuous", "Once"}."Once", "VISA session"=w288) -> ("error out"=w282:errorcluster)  [unwired: 8 out]
      }
      event #9 {
        n217 = event-data() -> ()  [unwired: 7 out]
        n218 = local read "Ch1 NOT Toggle"() -> (w304:bool)
        n219 = local read "Ch2 NOT Toggle"() -> (w303:bool)
        n220 = local read "Ch2 Toggle"() -> (w298:bool)
        n221 = local read "Ch1 Toggle"() -> (w300:bool)
        n222 = local read "Ch1 Sync"() -> (w306:bool)
        n223 = local read "Ch2 Sync"() -> (w305:bool)
        n224 = case shown="True" w306 {
          tunnel: [w309 w310] -> w299
          tunnel: w304 -> [w309 _]
          tunnel: w300 -> [_ w310]
          frame #0 {
          }
          frame #1 {
            n225 = local write "Ch1 NOT Toggle"(w310) -> ()
          }
        }
        n226 = case shown="True" w305 {
          tunnel: [w307 w308] -> w297
          tunnel: w303 -> [w307 _]
          tunnel: w298 -> [_ w308]
          frame #0 {
          }
          frame #1 {
            n227 = local write "Ch2 NOT Toggle"(w308) -> ()
          }
        }
        n228 = call "HP81110A Output Set - Fast.vi"("notoutput2"=w297, "output1"=w300, "error in (no error)"=w295, "output2"=w298, "notoutput1"=w299, "VISA session"=w296) -> ("error out"=w294:errorcluster)  [unwired: 5 out]
        n229 = Build Array(w300, w299, w298, w297) -> (w301:bool[])
        n230 = Bundle By Name(cluster=w293, "Outputs 1/!1/2/!2"=w301) -> (w302:T3)
      }
      event #10 {
        n231 = event-data() -> ("NewVal"=w311:dbl[unit])  [unwired: 6 out]
        n232 = Reciprocal(x=w311) -> (1/x=w316:dbl[unit])
        n233 = local write "OverallFreqSet"(w316) -> ()
        n234 = local read "Width/Duty\nUP/DOWN Ch2"() -> (w312:bool)
        n235 = local read "Width/Duty\nUP/DOWN Ch1"() -> (w313:bool)
        n236 = case shown="True" w313 {
          tunnel: w311 -> [w329 w332]
          frame #0 {
            n237 = local read "Ch1Duty (%) Set"() -> (w327:dbl)
            n238 = Divide(x=w327, y=100.0) -> (x/y=w330:dbl)
            n239 = Multiply(x=w330, y=w329) -> (x*y=w328:dbl[unit])
            n240 = local write "Ch1Width"(w328) -> ()
          }
          frame #1 {
            n241 = local read "Ch1Width"() -> (w333:dbl[unit])
            n242 = Divide(x=w333, y=w332) -> (x/y=w336:dbl)
            n243 = Multiply(x=w336, y=100) -> (x*y=w335:dbl)
            n244 = local write "Ch1Duty (%) Set"(w335) -> ()
          }
        }
        n245 = case shown="True" w312 {
          tunnel: w311 -> [w318 w326]
          frame #0 {
            n246 = local read "Ch2Duty (%) Set"() -> (w321:dbl)
            n247 = Divide(x=w321, y=100.0) -> (x/y=w320:dbl)
            n248 = Multiply(x=w320, y=w318) -> (x*y=w317:dbl[unit])
            n249 = local write "Ch2Width"(w317) -> ()
          }
          frame #1 {
            n250 = local read "Ch2Width"() -> (w325:dbl[unit])
            n251 = Divide(x=w325, y=w326) -> (x/y=w324:dbl)
            n252 = Multiply(x=w324, y=100) -> (x*y=w322:dbl)
            n253 = local write "Ch2Duty (%) Set"(w322) -> ()
          }
        }
      }
      event #11 {
        n254 = event-data() -> ("NewVal"=w348:dbl[unit])  [unwired: 6 out]
        n255 = local read "Ch1Width"() -> (w347:dbl[unit])
        n256 = local read "Ch2Width"() -> (w346:dbl[unit])
        n257 = Reciprocal(x=w348) -> (1/x=w345:dbl[unit])
        n258 = Divide(x=w347, y=w345) -> (x/y=w342:dbl)
        n259 = Divide(x=w346, y=w345) -> (x/y=w340:dbl)
        n260 = local write "OverallPeriodSet"(w345) -> ()
        n261 = Multiply(x=w342, y=100) -> (x*y=w341:dbl)
        n262 = Multiply(x=w340, y=100) -> (x*y=w339:dbl)
        n263 = local write "Ch1Duty (%) Set"(w341) -> ()
        n264 = local write "Ch2Duty (%) Set"(w339) -> ()
      }
      event #12 {
        n265 = event-data() -> ()  [unwired: 7 out]
      }
      event #13 {
        n266 = event-data() -> ()  [unwired: 7 out]
        n267 = local read "Width/Duty\nUP/DOWN Ch1"() -> (w361:bool)
        n268 = local read "Width/Duty\nUP/DOWN Ch2"() -> (w358:bool)
        n269 = local read "Width/Duty\nUP/DOWN Ch1"() -> (w359:bool)
        n270 = local read "Width/Duty\nUP/DOWN Ch2"() -> (w360:bool)
        n271 = Bundle By Name(cluster=w357, "Ch1Width(true)"=w359, "Ch2Width(true)"=w358) -> (w356:T3)
        n272 = Select(t=2, s=w361, f=0) -> (s? t:f=w352:i32)
        n273 = Select(t=2, s=w360, f=0) -> (s? t:f=w353:i32)
        n274 = Select(t=0, s=w358, f=2) -> (s? t:f=w354:i32)
        n275 = Select(t=0, s=w359, f=2) -> (s? t:f=w355:i32)
        n276 = property on="Ch1Duty (%) Set" class="DigNum (strict)"("Disabled"=w352) -> ()  [unwired: 2 in, 2 out]
        n277 = property on="Ch2Duty (%) Set" class="DigNum (strict)"("Disabled"=w353) -> ()  [unwired: 2 in, 2 out]
        n278 = property on="Ch2WidthSet" class="DigNum (strict)"("DisabledEnum"=w354) -> ()  [unwired: 2 in, 2 out]
        n279 = property on="Ch1WidthSet" class="DigNum (strict)"("DisabledEnum"=w355) -> ()  [unwired: 2 in, 2 out]
        n280 = property on="Ch2Duty (%)" class="DigNum (strict)"("Disabled"=w353) -> ()  [unwired: 2 in, 2 out]
        n281 = property on="Ch2Width" class="DigNum (strict)"("DisabledEnum"=w354) -> ()  [unwired: 2 in, 2 out]
        n282 = property on="Ch1Width" class="DigNum (strict)"("DisabledEnum"=w355) -> ()  [unwired: 2 in, 2 out]
        n283 = property on="Ch1Duty (%)" class="DigNum (strict)"("Disabled"=w352) -> ()  [unwired: 2 in, 2 out]
      }
      event #14 {
        # "this hard codes to have the duty cycle be read as a width"
        n284 = event-data() -> ()  [unwired: 7 out]
        n285 = local read "Ch1WidthSet"() -> (w375:dbl[unit])
        n286 = local read "Ch1Duty (%) Set"() -> (w379:dbl)
        n287 = local read "OverallPeriodSet"() -> (w377:dbl[unit])
        n288 = local read "Width/Duty\nUP/DOWN Ch1"() -> (w374:bool)
        n289 = Divide(x=w379, y=100.0) -> (x/y=w378:dbl)
        n290 = Multiply(x=w378, y=w377) -> (x*y=w376:dbl[unit])
        n291 = Select(t=w375, s=w374, f=w376) -> (s? t:f=w373:dbl[unit])
        n292 = local write "Ch1WidthSet"(w373) -> ()
      }
      event #15 {
        # "this hard codes to have the duty cycle be read as a width"
        n293 = event-data() -> ()  [unwired: 7 out]
        n294 = local read "Ch2WidthSet"() -> (w384:dbl[unit])
        n295 = local read "Ch2Duty (%) Set"() -> (w390:dbl)
        n296 = local read "OverallPeriodSet"() -> (w387:dbl[unit])
        n297 = local read "Width/Duty\nUP/DOWN Ch2"() -> (w385:bool)
        n298 = Divide(x=w390, y=100.0) -> (x/y=w388:dbl)
        n299 = Multiply(x=w388, y=w387) -> (x*y=w386:dbl[unit])
        n300 = Select(t=w384, s=w385, f=w386) -> (s? t:f=w383:dbl[unit])
        n301 = local write "Ch2WidthSet"(w383) -> ()
      }
      event #16 {
        n302 = event-data() -> ("NewVal"=w397:dbl[unit])  [unwired: 6 out]
        n303 = local read "OverallPeriodSet"() -> (w396:dbl[unit])
        n304 = Divide(x=w397, y=w396) -> (x/y=w395:dbl)
        n305 = Multiply(x=100, y=w395) -> (x*y=w393:dbl)
        n306 = local write "Ch1Duty (%) Set"(w393) -> ()
      }
      event #17 {
        n307 = event-data() -> ("NewVal"=w400:dbl[unit])  [unwired: 6 out]
        n308 = local read "OverallPeriodSet"() -> (w404:dbl[unit])
        n309 = Divide(x=w400, y=w404) -> (x/y=w403:dbl)
        n310 = Multiply(x=100, y=w403) -> (x*y=w401:dbl)
        n311 = local write "Ch2Duty (%) Set"(w401) -> ()
      }
    }
    n312 = call "HP81110A Error Query.vi"("VISA session"=w24, "error in (no error)"=w23) -> ("error out"=w28:errorcluster)  [unwired: 13 out]
    n313 = call <vilib>:"Simple Error Handler.vi"("error in (no error)"=w28) -> ("error out"=w18:errorcluster)  [unwired: 1 in, 7 out]
  }
  "error out" <- w6
